vi "SEND WRITE PORT.vi"(8 "error in (no error)":errorcluster, 10 "CANAL":u8, 11 "SERIAL DEVICE in":refnum<class "SERIAL DEVICE.lvclass">) -> (0 "error out":errorcluster, 2 "read buffer":string, 3 "SERIAL DEVICE out":refnum<class "SERIAL DEVICE.lvclass">)   [LabVIEW 2019, in "SERIAL DEVICE.lvclass"]
uses:
  SERIAL DEVICE.lvclass
  SERIAL DEVICE.lvclass/SERIAL DEVICE.ctl
  9f88877d-c6d6-43aa-9861-71a693b3c7d2.vi
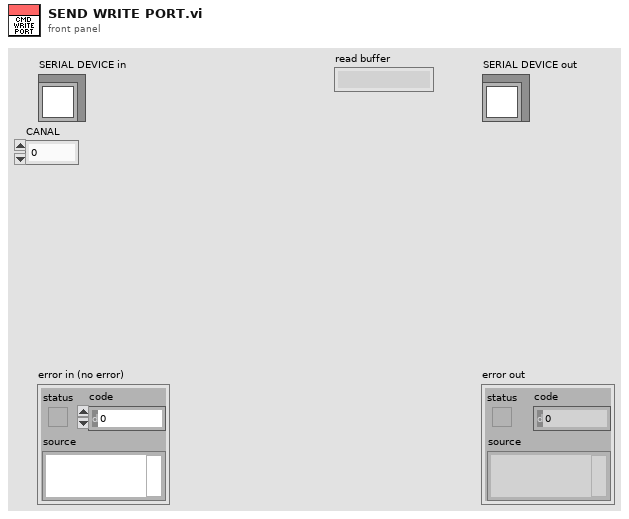
[diagram p1: front panel]
types:
  T1 = typedef "MICROS.ctl" = string
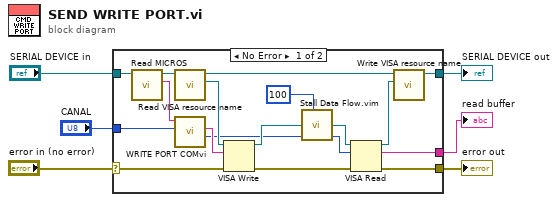
[diagram p0: block diagram]
diagram:
  n1 = case shown="No Error" "error in (no error)" {
    selector: "error in (no error)" -> [w14 w25]
    tunnel: [w13 w25] -> w5
    tunnel: [w16 w24] -> w3
    tunnel: "SERIAL DEVICE in" -> [w23 w24]
    tunnel: "CANAL" -> [w10 _]
    tunnel: [w19 _] -> w1
    frame No Error {
      n2 = call "Read MICROS.vi"("SERIAL DEVICE in"=w23) -> ("MICROS"=w9:T1, "SERIAL DEVICE out"=w12:refnum<class "SERIAL DEVICE.lvclass">)  [unwired: 8 in, 1 out]
      n3 = call "Read VISA resource name.vi"("SERIAL DEVICE in"=w12) -> ("VISA resource name"=w22:refnum<visa-resource-name>, "SERIAL DEVICE out"=w17:refnum<class "SERIAL DEVICE.lvclass">)  [unwired: 8 in, 1 out]
      n4 = call "WRITE PORT COMvi.vi"("CANAL"=w10, "MICROS"=w9) -> ("BYTES EXPECTED"=w7:i32, "COMANDO"=w8:string)  [unwired: 7 in, 1 out]
      n5 = VISA Write(VISA resource name=w22, write buffer=w8, error in (no error)=w14) -> (VISA resource name out=w21:refnum<visa-resource-name>, error out=w15:errorcluster)  [unwired: 1 out]
      n6 = call "Stall Data Flow.vim"("value in"=w21, "milliseconds to wait"=u32 100) -> ("value out"=w20:refnum<visa-resource-name>)  [unwired: 1 out]
      n7 = VISA Read(VISA resource name=w20, byte count=w7, error in (no error)=w15) -> (VISA resource name out=w18:refnum<visa-resource-name>, read buffer=w19:string, error out=w13:errorcluster)  [unwired: 1 out]
      n8 = call "Write VISA resource name.vi"("VISA resource name"=w18, "SERIAL DEVICE in"=w17) -> ("SERIAL DEVICE out"=w16:refnum<class "SERIAL DEVICE.lvclass">)  [unwired: 8 in, 1 out]
    }
    frame Error {
    }
  }
  "error out" <- w5
  "SERIAL DEVICE out" <- w3
  "read buffer" <- w1
